vi "UI Framework.vi"() -> ()   [LabVIEW 2013]
uses:
  Controllers/Main UI Controller/Main UI Controller.lvclass
  <vilib>/Utility/miscctls.llb/LVPositionTypeDef.ctl
  <vilib>/ActorFramework/Message Queue/Message Queue.lvclass/Message Queue.ctl
  <vilib>/ActorFrameworkMVC/UI Controller Messages/Set Subpanel Msg/Set Subpanel Msg.lvclass/Set Subpanel Msg.ctl
  <vilib>/ActorFramework/Message Enqueuer/Message Enqueuer.lvclass/Message Enqueuer.ctl
  <vilib>/ActorFrameworkMVC/UI Controller Messages/Move Subpanel Msg/Move Subpanel Msg.lvclass/Move Subpanel Msg.ctl
  <vilib>/ActorFrameworkMVC/UI Controller Messages/Set Splitter Msg/Set Splitter Msg.lvclass/Set Splitter Msg.ctl
  <vilib>/ActorFrameworkMVC/UI Controller Messages/Move Splitter Msg/Move Splitter Msg.lvclass/Move Splitter Msg.ctl
  <vilib>/ActorFrameworkMVC/UI Controller Messages/Insert Subpanel Msg/Insert Subpanel Msg.lvclass/Insert Subpanel Msg.ctl
  <vilib>/ActorFramework/Message Enqueuer/Enqueue.vi
  <vilib>/ActorFramework/Message Priority Queue/Priority Enqueue.vi
  <vilib>/ActorFrameworkMVC/UI Controller Messages/Set Subpanel Msg/Set Subpanel Msg.lvclass
  <vilib>/ActorFrameworkMVC/UI Controller Messages/Move Subpanel Msg/Move Subpanel Msg.lvclass
  <vilib>/ActorFrameworkMVC/UI Controller Messages/Set Splitter Msg/Set Splitter Msg.lvclass
  <vilib>/ActorFrameworkMVC/UI Controller Messages/Move Splitter Msg/Move Splitter Msg.lvclass
  Models/Main Model Messages/List Project File Msg/List Project File Msg.lvclass
  Models/Main Model Messages/Update Project Number Msg/Update Project Number Msg.lvclass
  Models/Main Model Messages/List Sensor File Msg/List Sensor File Msg.lvclass
  Models/Main Model Messages/Update Sensor Number Msg/Update Sensor Number Msg.lvclass
  <vilib>/ActorFrameworkMVC/UI Controller Messages/Insert Subpanel Msg/Insert Subpanel Msg.lvclass
  <vilib>/ActorFramework/Stop Msg/Stop Msg.lvclass
  <vilib>/ActorFramework/Message Queue/Message Queue.lvclass
  <vilib>/ActorFramework/Actor/Actor.lvclass
  <vilib>/ActorFrameworkMVC/UI Controller Messages/Get Model Actor Enqueuer Msg/Get Model Actor Enqueuer Msg.lvclass
panel:
  in  "Exit":bool
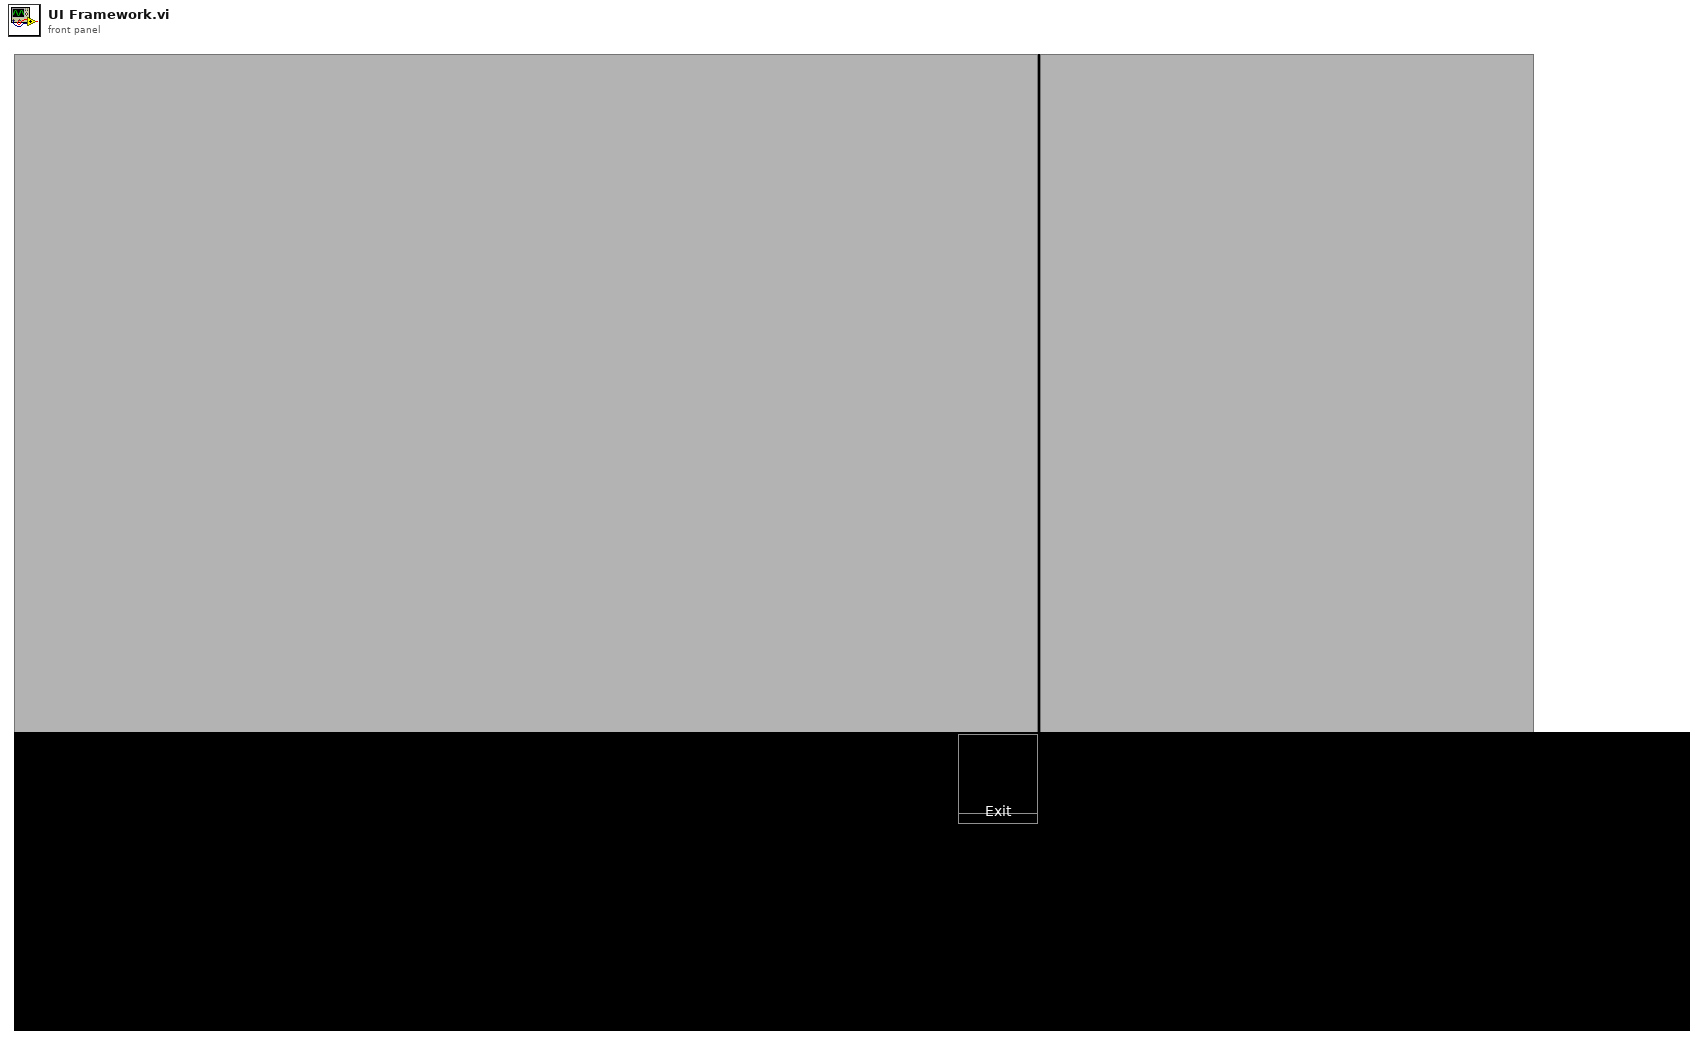
[diagram p1: front panel]
types:
  T1 = typedef "LVPositionTypeDef.ctl" = cluster{"Left":i32, "Top":i32}
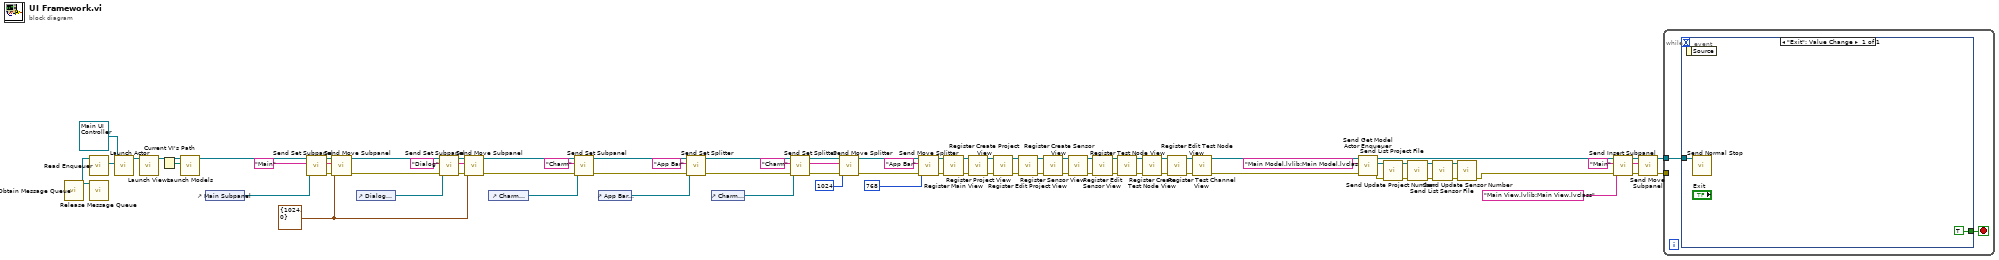
[diagram p0: block diagram]
diagram:
  w37 = T1 {"Left"=1024, "Top"=0} ("Position (0,0)")
  w46 = "Main" ("Subpanel Name")
  w34 = "Charm" ("Splitter Name")
  w38 = "Dialog" ("Subpanel Name")
  w40 = "Main" ("Subpanel Name")
  n1 = call <vilib>:"Obtain Message Queue.vi"() -> ("Message Queue"=w66:refnum<class "Message Queue.lvclass">)  [unwired: 10 in, 1 out]
  n2 = call <vilib>:"Read Enqueuer.vi"("Message Queue"=w66) -> ("Message Enqueuer"=w67:refnum<class "Message Enqueuer.lvclass">)  [unwired: 10 in]
  n3 = call <vilib>:"Release Message Queue.vi"("Message Queue"=w66) -> ()  [unwired: 9 in, 2 out]
  n4 = call <vilib>:"Launch Actor.vi"("Actor-to-Caller Enqueuer"=w67, "Actor"=refnum<class "Main UI Controller.lvclass"> refnum ("Main UI Controller.lvlib:Main UI Controller.lvclass")) -> ("Caller-To-Actor Enqueuer"=w12:refnum<class "Message Enqueuer.lvclass">)  [unwired: 8 in, 1 out]
  n5 = call "Launch Views.vi"("Message Enqueuer in"=w12) -> ("Message Enqueuer out"=w11:refnum<class "Message Enqueuer.lvclass">)  [unwired: 10 in]
  n6 = Current VI's Path() -> (path=w13:path)
  n7 = call "Launch Models.vi"("Top Level Path"=w13, "Message Enqueuer in"=w11) -> ("Message Enqueuer out"=w10:refnum<class "Message Enqueuer.lvclass">)  [unwired: 9 in]
  n8 = control-ref of="Main Subpanel"() -> (w42:refnum<vi>)
  n9 = call <vilib>:"Send Set Subpanel.vi"("SubPanel Reference"=w42, "Subpanel Name"=w40, "Message Enqueuer"=w10) -> ("error out"=w14:errorcluster, "Message Enqueuer out"=w63:refnum<class "Message Enqueuer.lvclass">)  [unwired: 7 in]
  n10 = call <vilib>:"Send Move Subpanel.vi"("error in (no error)"=w14, "Position (0,0)"=w37, "Subpanel Name"=w40, "Message Enqueuer"=w63) -> ("error out"=w28:errorcluster, "Message Enqueuer out"=w41:refnum<class "Message Enqueuer.lvclass">)  [unwired: 6 in]
  n11 = control-ref of="Dialog Subpanel"() -> (w61:refnum<vi>)
  n12 = call <vilib>:"Send Set Subpanel.vi"("error in (no error)"=w28, "SubPanel Reference"=w61, "Subpanel Name"=w38, "Message Enqueuer"=w41) -> ("error out"=w27:errorcluster, "Message Enqueuer out"=w62:refnum<class "Message Enqueuer.lvclass">)  [unwired: 6 in]
  n13 = call <vilib>:"Send Move Subpanel.vi"("error in (no error)"=w27, "Position (0,0)"=w37, "Subpanel Name"=w38, "Message Enqueuer"=w62) -> ("error out"=w26:errorcluster, "Message Enqueuer out"=w39:refnum<class "Message Enqueuer.lvclass">)  [unwired: 6 in]
  n14 = control-ref of="Charm Subpanel"() -> (w60:refnum<vi>)
  n15 = call <vilib>:"Send Set Subpanel.vi"("error in (no error)"=w26, "SubPanel Reference"=w60, "Subpanel Name"="Charm", "Message Enqueuer"=w39) -> ("error out"=w25:errorcluster, "Message Enqueuer out"=w59:refnum<class "Message Enqueuer.lvclass">)  [unwired: 6 in]
  n16 = control-ref of="App Bar Splitter"() -> (w56:refnum<vi>)
  n17 = call <vilib>:"Send Set Splitter.vi"("error in (no error)"=w25, "Splitter Reference"=w56, "Splitter Name"="App Bar", "Message Enqueuer"=w59) -> ("error out"=w24:errorcluster, "Message Enqueuer out"=w57:refnum<class "Message Enqueuer.lvclass">)  [unwired: 6 in]
  n18 = control-ref of="Charm Splitter"() -> (w55:refnum<vi>)
  n19 = call <vilib>:"Send Set Splitter.vi"("error in (no error)"=w24, "Splitter Reference"=w55, "Splitter Name"=w34, "Message Enqueuer"=w57) -> ("error out"=w23:errorcluster, "Message Enqueuer out"=w54:refnum<class "Message Enqueuer.lvclass">)  [unwired: 6 in]
  n20 = call <vilib>:"Send Move Splitter.vi"("error in (no error)"=w23, "Splitter Position"=1024, "Splitter Name"=w34, "Message Enqueuer"=w54) -> ("error out"=w22:errorcluster, "Message Enqueuer out"=w35:refnum<class "Message Enqueuer.lvclass">)  [unwired: 6 in]
  n21 = call <vilib>:"Send Move Splitter.vi"("error in (no error)"=w22, "Splitter Position"=768, "Splitter Name"="App Bar", "Message Enqueuer"=w35) -> ("error out"=w21:errorcluster, "Message Enqueuer out"=w32:refnum<class "Message Enqueuer.lvclass">)  [unwired: 6 in]
  n22 = call "Register Main View.vi"("Message Enqueuer in"=w32) -> ("Message Enqueuer out"=w36:refnum<class "Message Enqueuer.lvclass">)  [unwired: 10 in]
  n23 = call "Register Project View.vi"("Message Enqueuer in"=w36) -> ("Message Enqueuer out"=w29:refnum<class "Message Enqueuer.lvclass">)  [unwired: 10 in]
  n24 = call "Register Create Project View.vi"("Message Enqueuer in"=w29) -> ("Message Enqueuer out"=w9:refnum<class "Message Enqueuer.lvclass">)  [unwired: 10 in]
  n25 = call "Register Edit Project View.vi"("Message Enqueuer in"=w9) -> ("Message Enqueuer out"=w8:refnum<class "Message Enqueuer.lvclass">)  [unwired: 10 in]
  n26 = call "Register Sensor View.vi"("Message Enqueuer in"=w8) -> ("Message Enqueuer out"=w7:refnum<class "Message Enqueuer.lvclass">)  [unwired: 10 in]
  n27 = call "Register Create Sensor View.vi"("Message Enqueuer in"=w7) -> ("Message Enqueuer out"=w6:refnum<class "Message Enqueuer.lvclass">)  [unwired: 10 in]
  n28 = call "Register Edit Sensor View.vi"("Message Enqueuer in"=w6) -> ("Message Enqueuer out"=w5:refnum<class "Message Enqueuer.lvclass">)  [unwired: 10 in]
  n29 = call "Register Test Node View.vi"("Message Enqueuer in"=w5) -> ("Message Enqueuer out"=w4:refnum<class "Message Enqueuer.lvclass">)  [unwired: 10 in]
  n30 = call "Register Create Test Node View.vi"("Message Enqueuer in"=w4) -> ("Message Enqueuer out"=w3:refnum<class "Message Enqueuer.lvclass">)  [unwired: 10 in]
  n31 = call "Register Edit Test Node View.vi"("Message Enqueuer in"=w3) -> ("Message Enqueuer out"=w2:refnum<class "Message Enqueuer.lvclass">)  [unwired: 10 in]
  n32 = call "Register Test Channel View.vi"("Message Enqueuer in"=w2) -> ("Message Enqueuer out"=w1:refnum<class "Message Enqueuer.lvclass">)  [unwired: 10 in]
  n33 = call <vilib>:"Send Get Model Actor Enqueuer.vi"("error in (no error)"=w21, "Model Name"="Main Model.lvlib:Main Model.lvclass", "Message Enqueuer in"=w1) -> ("error out"=w20:errorcluster, "Reply"=w51:refnum<class "Message Enqueuer.lvclass">, "Message Enqueuer out"=w52:refnum<class "Message Enqueuer.lvclass">)  [unwired: 5 in, 1 out]
  n34 = call "Send List Project File.vi"("error in (no error)"=w20, "Message Enqueuer"=w51) -> ("error out"=w19:errorcluster, "Message Enqueuer out"=w50:refnum<class "Message Enqueuer.lvclass">)  [unwired: 8 in]
  n35 = call "Send Update Project Number.vi"("error in (no error)"=w19, "Message Enqueuer"=w50) -> ("error out"=w18:errorcluster, "Message Enqueuer out"=w44:refnum<class "Message Enqueuer.lvclass">)  [unwired: 8 in]
  n36 = call "Send List Sensor File.vi"("error in (no error)"=w18, "Message Enqueuer"=w44) -> ("error out"=w17:errorcluster, "Message Enqueuer out"=w43:refnum<class "Message Enqueuer.lvclass">)  [unwired: 8 in]
  n37 = call "Send Update Sensor Number.vi"("error in (no error)"=w17, "Message Enqueuer"=w43) -> ("error out"=w45:errorcluster)  [unwired: 8 in, 1 out]
  n38 = call <vilib>:"Send Insert Subpanel.vi"("error in (no error)"=w45, "View Name"="Main View.lvlib:Main View.lvclass", "Subpanel Name"=w46, "Message Enqueuer"=w52) -> ("error out"=w16:errorcluster, "Message Enqueuer out"=w49:refnum<class "Message Enqueuer.lvclass">)  [unwired: 6 in]
  n39 = call <vilib>:"Send Move Subpanel.vi"("error in (no error)"=w16, "Subpanel Name"=w46, "Message Enqueuer"=w49) -> ("error out"=w15:errorcluster, "Message Enqueuer out"=w47:refnum<class "Message Enqueuer.lvclass">)  [unwired: 7 in]
  n40 = while {
    tunnel: w47 -> [w68]
    tunnel: w15 -> [_]
    stop <- w69 stop-if-true
    n41 = event shown="[0] \"Exit\": Value Change" {
      selector: _ -> [_]
      dyn-events: _ -> [_]
      timeout: _ -> [_]
      tunnel: [TRUE] -> w69
      tunnel: w68 -> [w70]
      event "Exit": Value Change {
        n42 = event-data() -> ()  [unwired: 1 in, 1 out]
        n43 = call <vilib>:"Send Normal Stop.vi"("Message Enqueuer"=w70) -> ()  [unwired: 10 in, 1 out]
      }
    }
  }
